vi "Measurement UI.vi"() -> ()   [LabVIEW 2021, in "Efficiency_Channel Ganging_UI.lvlib"]
uses:
  Efficiency_Channel Ganging_UI.lvlib
panel:
  in  "MeasGraphs":enum32{"Efficiency", "Hidden Controls"}(tab)
  out "EfficiencyGraph":T1(graph)
  in  "Load current pole-zero ratios":dbl[](array[numeric])
  in  "Load current compensation frequencies":dbl[](array[numeric])
  in  "Load current gain bandwidths":dbl[](array[numeric])
  in  "Source voltage pole-zero ratios":dbl[](array[numeric])
  in  "Source voltage compensation frequencies":dbl[](array[numeric])
  in  "Source voltage gain bandwidths":dbl[](array[numeric])
  in  "Load slave resource names":string[](array[string])
  in  "Load master resource name":string
  in  "Source slave resource names":string[](array[string])
  in  "Source master resource name":string
  out "Load sweep points":i32
  out "Source sweep points":i32
  out "Voltage values":dbl[](array[numeric])
  out "Efficiency":dbl[](array[numeric])
  out "Ganged load currents":dbl[](array[numeric])
  in  "MeasConfigurations":T2(tab)=enum."Source Config"
  in  "Source delay":dbl=0.005 caption="SOURCE DELAY" format="%.3ps"
  in  "DUT setup time":dbl=1.0 caption="DUT SETUP TIME" format="%.3ps"
  in  "Aperture time":dbl=0.005 caption="APERTURE TIME" format="%.3ps"
  in  "PPSSlaveResourceNames":refnum<k15>[](array[refnum]) caption="SLAVE RESOURCE NAMES"
  in  "PPSMasterResourceName":refnum<k15> caption="MASTER RESOURCE NAME"
  in  "Source stop voltage":dbl=14.0 caption="VOLTAGE STOP LEVEL" format="%#_6pV"
  in  "Source transient response":i32(ring)=1038 caption="TRANSIENT RESPONSE" items=["Slow"=1041, "Normal"=1038, "Fast"=1039, "Custom"=1042]
  in  "Source sense":i32(ring)=1009 caption="SENSE" items=["Local"=1008, "Remote"=1009]
  in  "Source voltage level range":dbl=20.0 caption="VOLTAGE LEVEL RANGE" format="%#_6pV"
  in  "Source start voltage":dbl=6.0 caption="VOLTAGE START LEVEL" format="%#_6pV"
  in  "Source current limit high":dbl=25.0 caption="CURRENT LIMIT/LIMIT HIGH" format="%#_6pA"
  in  "Source current limit range":dbl=25.0 caption="CURRENT LIMIT RANGE" format="%#_6pA"
  in  "Source limit symmetry":enum32{"Symmetric", "Asymmetric"}(ring)=enum."Asymmetric" caption="LIMIT SYMMETRY"
  in  "Source current limit low":dbl=-0.6 caption="CURRENT LIMIT LOW" format="%#_6pA"
  in  "Source system configuration":enum32{"Series", "Parallel"}(ring)=enum."Parallel" caption="SYSTEM CONFIG"
  in  "Source compliance":string="Compliance"
  in  "Source sourceadapt":string="SourceAdapt"
  in  "Source voltage sweep points":i32=4 caption="NO. OF POINTS"
  in  "Source Custom Transient Response":bool
  in  "Load current sweep points/points per decade":i32=10 caption="PTS/PTS PER DECADE"
  in  "Load sweep type":string(combo)="Logarithmic" caption="SWEEP TYPE"
  in  "Load stop current":dbl=50.0 caption="CURRENT STOP LEVEL" format="%#_6pA"
  in  "Load sourceadapt":string="SourceAdapt"
  in  "Load compliance":string="Compliance"
  in  "Load system configuration":enum32{"Series", "Parallel"}(ring)=enum."Parallel" caption="SYSTEM CONFIG"
  in  "Load voltage limit low":dbl caption="VOLTAGE  LIMIT LOW" format="%#_6pV"
  in  "Load limit symmetry":enum32{"Symmetric", "Asymmetric"}(ring) caption="LIMIT SYMMETRY"
  in  "Load voltage limit range":dbl=6.0 caption="VOLTAGE LIMIT RANGE" format="%#_6pV"
  in  "Load voltage limit high":dbl=inf caption="VOLTAGE LIMIT/LIMIT HIGH" format="%#_6p"
  in  "Load start current":dbl=2.0 caption="CURRENT START LEVEL" format="%#_6pA"
  in  "Load current level range":dbl=80.0 caption="CURRENT LEVEL RANGE" format="%#_6pA"
  in  "Load sense":i32(ring)=1009 caption="SENSE" items=["Local"=1008, "Remote"=1009]
  in  "Load transient response":i32(ring)=1038 caption="TRANSIENT RESPONSE" items=["Slow"=1041, "Normal"=1038, "Fast"=1039, "Custom"=1042]
  in  "LoadSlaveResourceNames":refnum<k15>[](array[refnum]) caption="SLAVE RESOURCE NAMES"
  in  "LoadMasterResourceName":refnum<k15> caption="MASTER RESOURCE NAME"
  in  "Load Custom Transient Response":bool
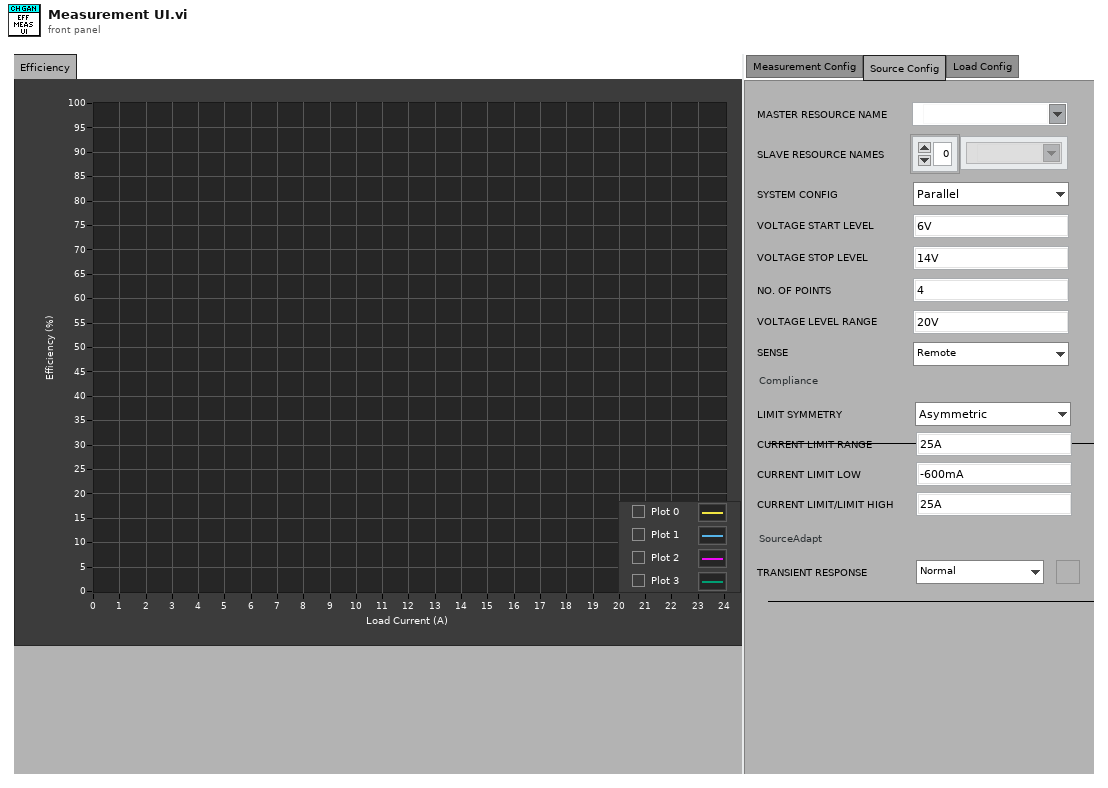
[diagram p1: front panel]
types:
  T1 = cluster{"Ganged load currents":dbl[], "Efficiency":dbl[]}[]
  T2 = enum32{"Measurement Config", "Source Config", "Load Config"}
  T3 = typedef "SourceAdapt Parameters.ctl" = cluster{"Voltage gain bandwidth":dbl, "Voltage compensation frequency":dbl, "Voltage pole-zero ratio":dbl, "Current gain bandwidth":dbl, "Current compensation frequency":dbl, "Current pole-zero ratio":dbl}[]
  T4 = cluster{"Ganged load currents":dbl[], "Efficiency":dbl[]}
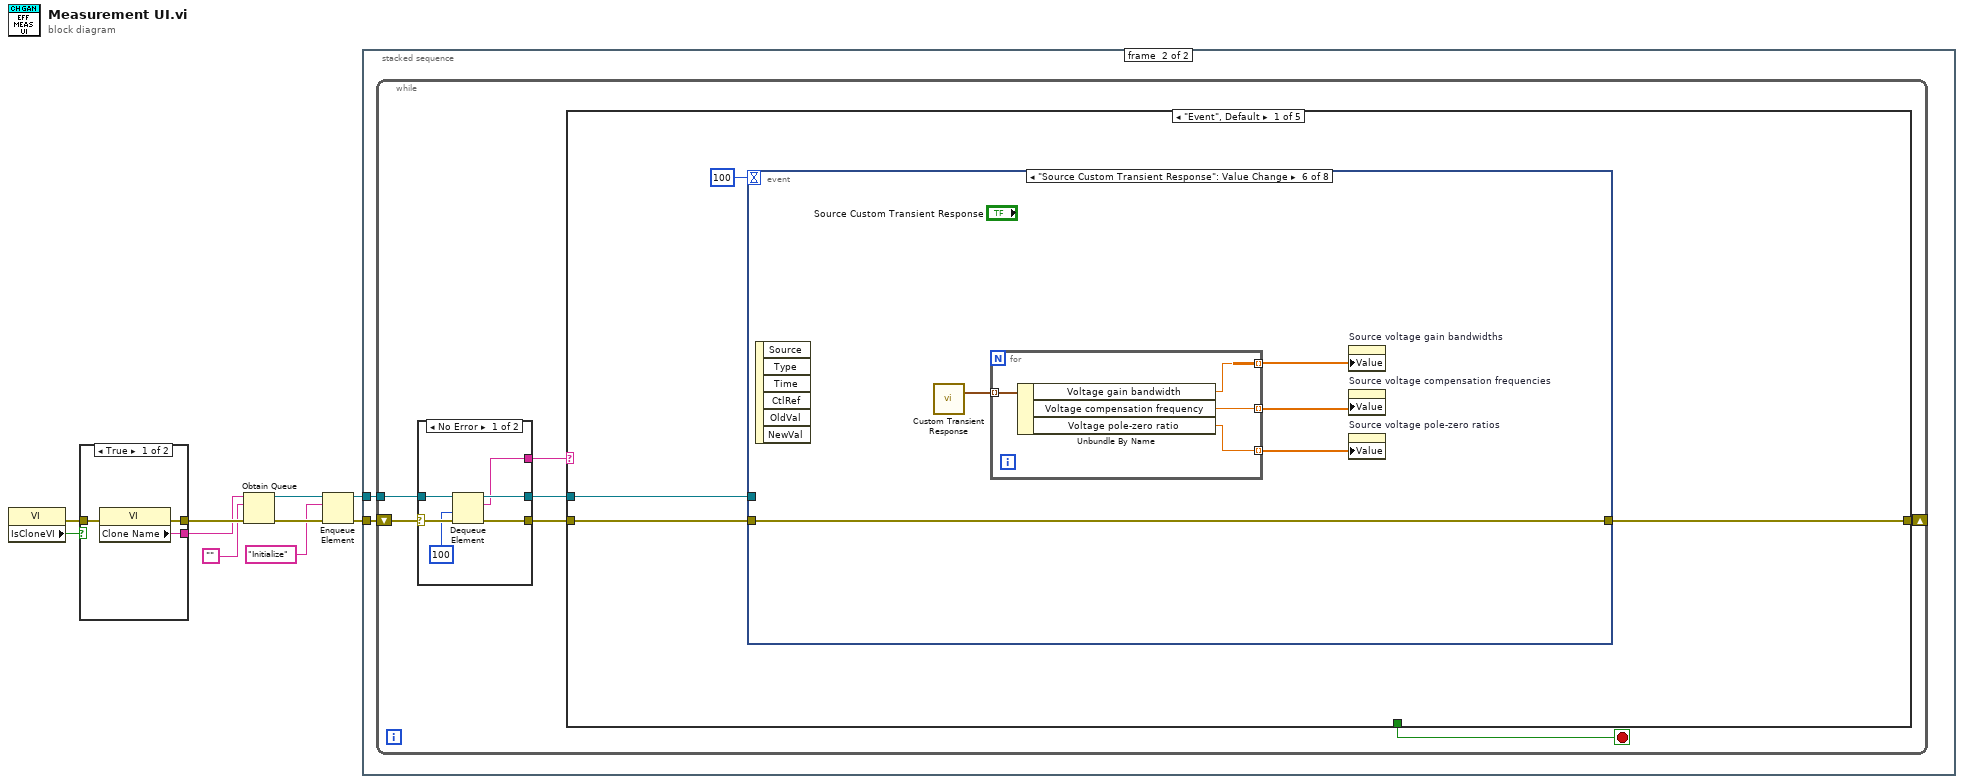
[diagram p0: block diagram]
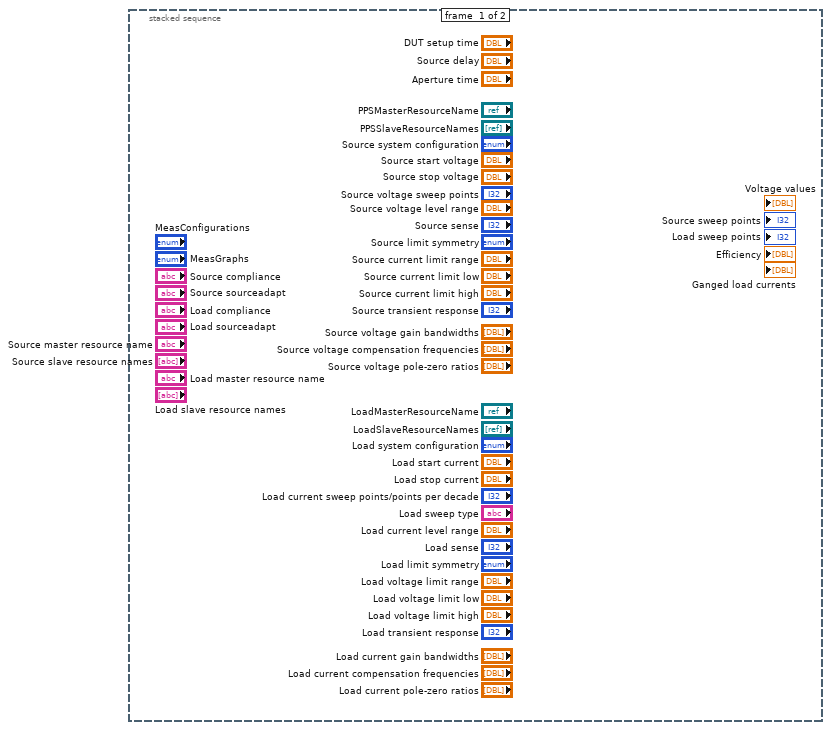
[diagram p2: hidden frame]
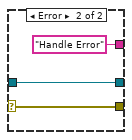
[diagram p3: hidden frame]
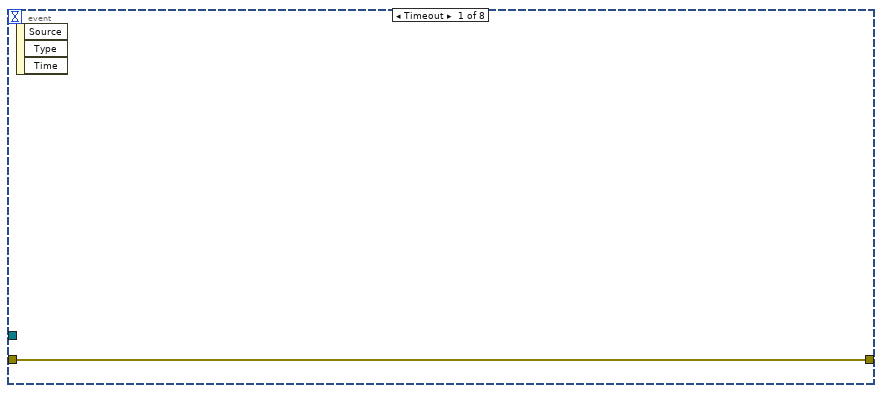
[diagram p4: hidden frame]
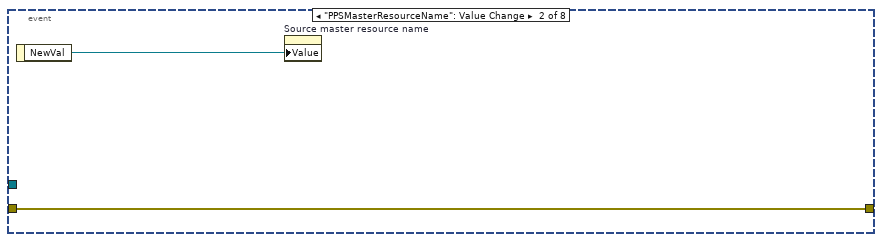
[diagram p5: hidden frame]
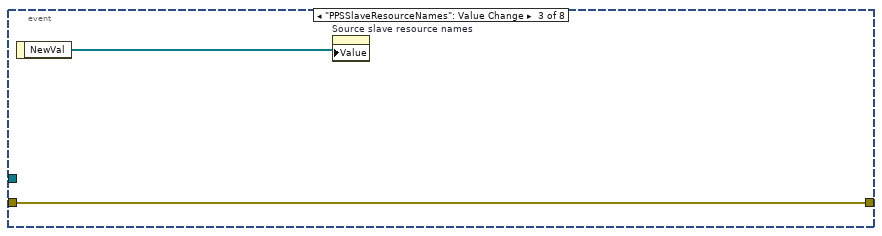
[diagram p6: hidden frame]
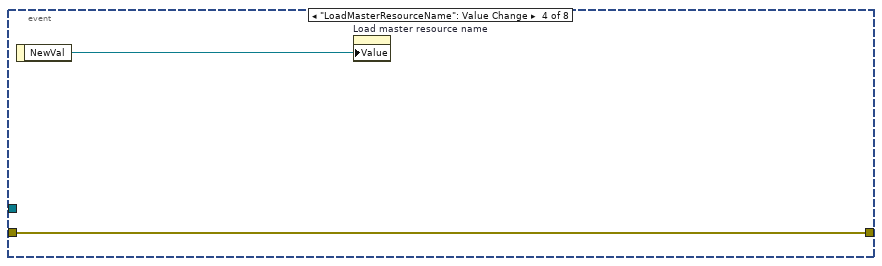
[diagram p7: hidden frame]
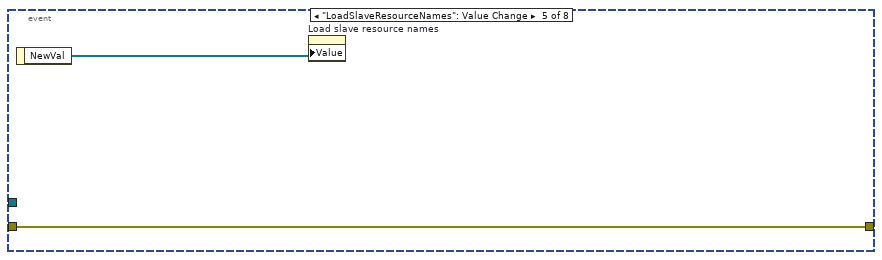
[diagram p8: hidden frame]
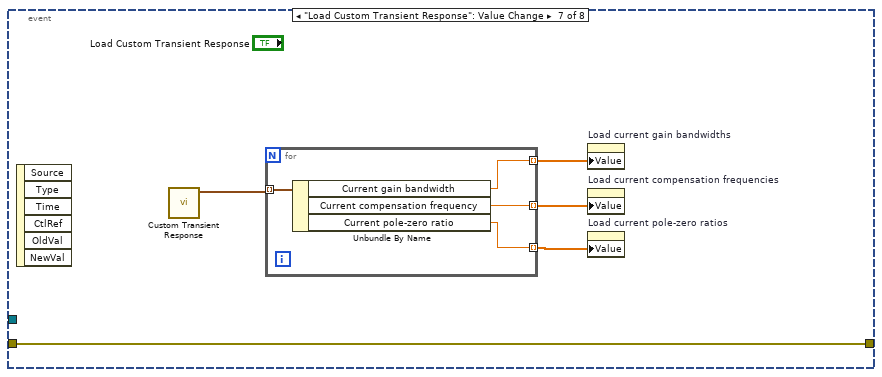
[diagram p9: hidden frame]
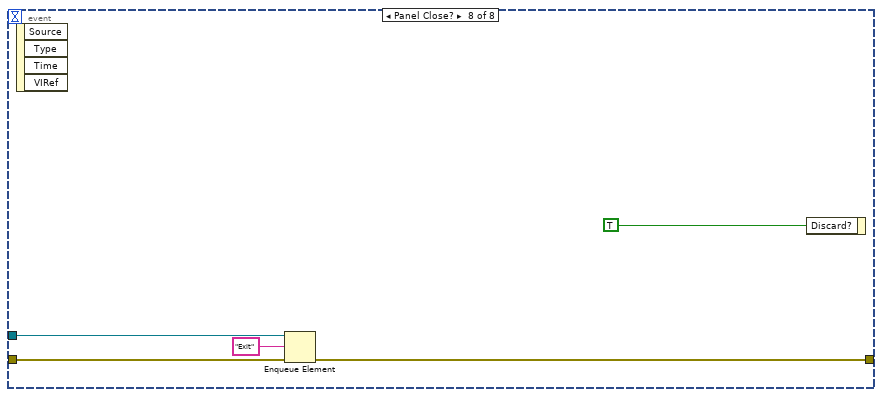
[diagram p10: hidden frame]
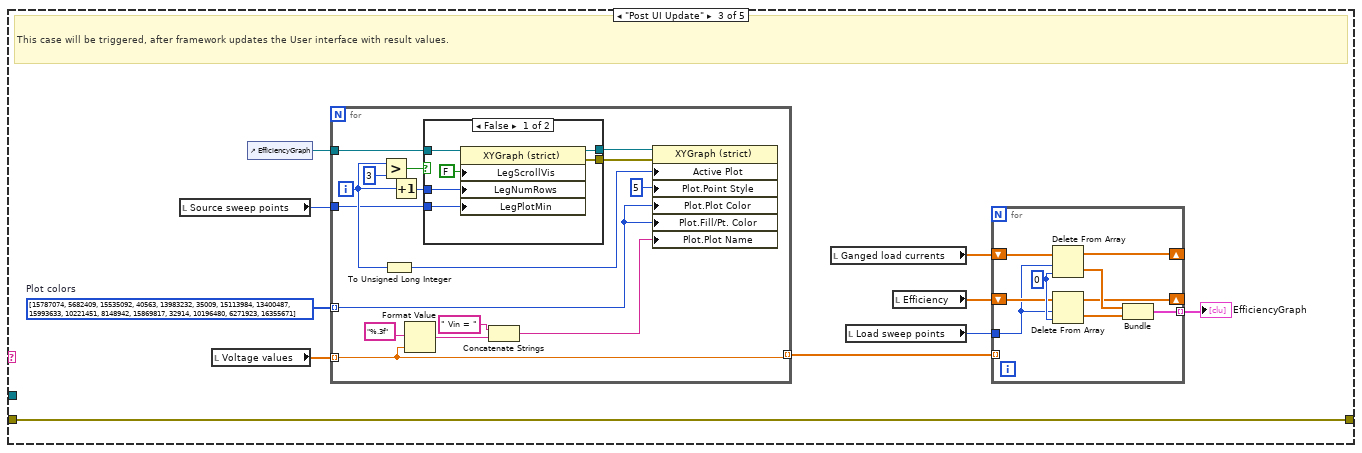
[diagram p12: hidden frame]
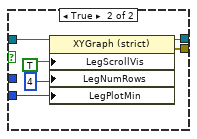
[diagram p13: hidden frame]
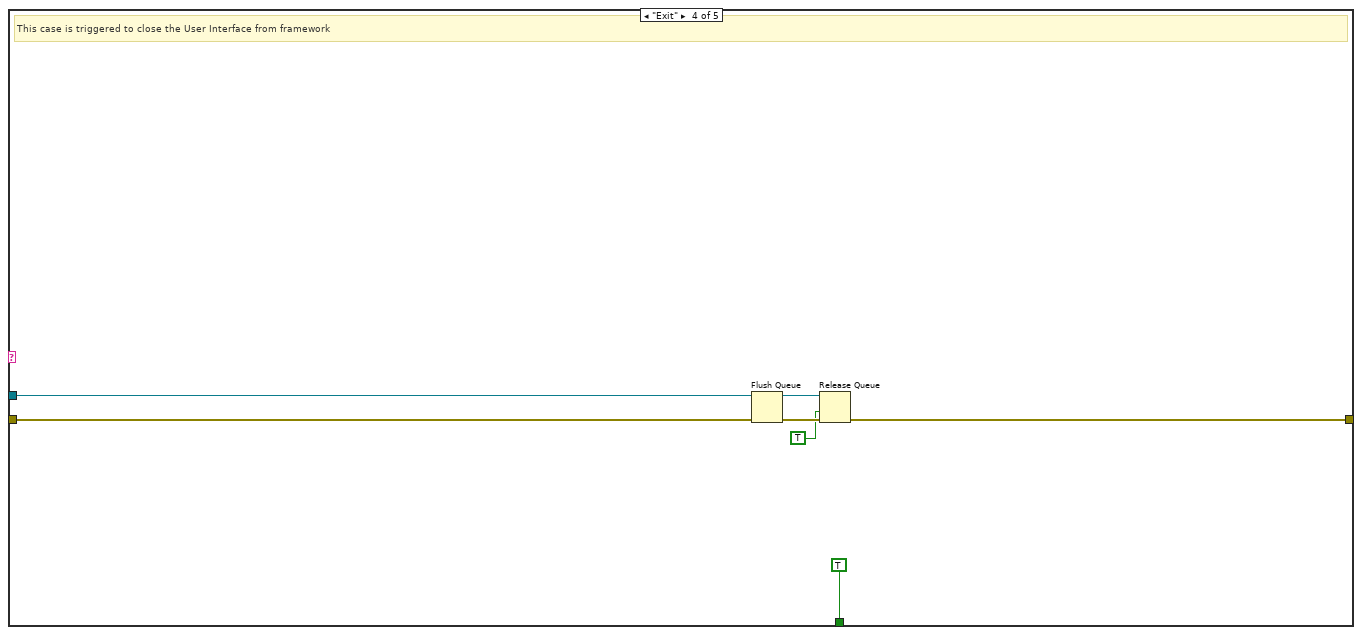
[diagram p14: hidden frame]
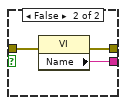
[diagram p16: hidden frame]
diagram:
  n1 = property class="VI"() -> (error out=w1:errorcluster, "IsCloneVI"=w2:bool)  [unwired: 2 in, 1 out]
  n2 = case shown="True" w2 {
    tunnel: [w13 w16] -> w10
    tunnel: [w12 w15] -> w9
    tunnel: w1 -> [w11 w14]
    frame True {
      n3 = property class="VI"(error in=w11) -> (error out=w13:errorcluster, "Clone Name"=w12:string)  [unwired: 1 in, 1 out]
    }
    frame False {
      n4 = property class="VI"(error in=w14) -> (error out=w16:errorcluster, "Name"=w15:string)  [unwired: 1 in, 1 out]
    }
  }
  n5 = Obtain Queue(name (unnamed)=w9, element data type="", error in (no error)=w10) -> (queue out=w6:refnum<queue>, error out=w8:errorcluster)  [unwired: 2 in, 1 out]
  n6 = Enqueue Element(queue=w6, element="Initialize", error in (no error)=w8) -> (queue out=w5:refnum<queue>, error out=w7:errorcluster)  [unwired: 1 in, 1 out]
  n7 = stacked-sequence {
    tunnel: w7 -> [_ w18]
    tunnel: w5 -> [_ w17]
    frame #0 {
    }
    frame #1 {
      n8 = while {
        shift-right: [w20] -> _
        shift-left: w18 -> [w25]
        tunnel: w17 -> [w23]
        stop <- w19 stop-if-true
        n9 = case shown="No Error" w25 {
          selector: w25 -> [w31 w34]
          tunnel: [w30 w34] -> w24
          tunnel: w23 -> [w29 w33]
          tunnel: [w28 w33] -> w22
          tunnel: [w27 "Handle Error"] -> w21
          frame No Error {
            n10 = Dequeue Element(queue=w29, timeout in ms (-1)=100, error in (no error)=w31) -> (queue out=w28:refnum<queue>, element=w27:string, error out=w30:errorcluster)  [unwired: 1 out]
          }
          frame Error {
          }
        }
        n11 = case shown="\"Event\", Default" w21 {
          tunnel: w24 -> [w37 w71 w81 w125 w126]
          tunnel: w22 -> [w35 _ _ w123 _]
          tunnel: [w38 w71 w81 w120 w126] -> w20
          tunnel: [_ _ _ TRUE _] -> w19
          frame "Event", Default {
            n12 = event shown="[5] \"Source Custom Transient Response\": Value Change" {
              selector: _ -> [_ _ _ _ _ _ _ _]
              dyn-events: _ -> [_ _ _ _ _ _ _ _]
              timeout: 100 -> [_ _ _ _ _ _ _ _]
              tunnel: [w39 w41 w43 w44 w46 w48 w57 w68] -> w38
              tunnel: w37 -> [w39 w41 w43 w44 w46 w48 w57 w69]
              tunnel: w35 -> [_ _ _ _ _ _ _ w67]
              event Timeout {
                n13 = event-data() -> ()  [unwired: 1 in, 3 out]
              }
              event "PPSMasterResourceName": Value Change {
                n14 = event-data() -> ("NewVal"=w40:refnum<k15>)  [unwired: 1 in]
                n15 = property on="Source master resource name" class="Str"("Value"=w40) -> ()  [unwired: 2 in, 2 out]
              }
              event "PPSSlaveResourceNames": Value Change {
                n16 = event-data() -> ("NewVal"=w42:refnum<k15>[])  [unwired: 1 in]
                n17 = property on="Source slave resource names" class="Arr (strict)"("Value"=w42) -> ()  [unwired: 2 in, 2 out]
              }
              event "LoadMasterResourceName": Value Change {
                n18 = event-data() -> ("NewVal"=w45:refnum<k15>)  [unwired: 1 in]
                n19 = property on="Load master resource name" class="Str"("Value"=w45) -> ()  [unwired: 2 in, 2 out]
              }
              event "LoadSlaveResourceNames": Value Change {
                n20 = event-data() -> ("NewVal"=w47:refnum<k15>[])  [unwired: 1 in]
                n21 = property on="Load slave resource names" class="Arr (strict)"("Value"=w47) -> ()  [unwired: 2 in, 2 out]
              }
              event "Source Custom Transient Response": Value Change {
                n22 = event-data() -> ()  [unwired: 1 in, 6 out]
                n23 = call "Custom Transient Response.vi"() -> ("SourceAdapt Parameters"=w52:T3)  [unwired: 11 in]
                n24 = for {
                  tunnel: w52 -> [w56] mode=indexing
                  tunnel: [w55] -> w51 mode=indexing
                  tunnel: [w54] -> w50 mode=indexing
                  tunnel: [w53] -> w49 mode=indexing
                  n25 = Unbundle By Name(w56) -> ("Voltage gain bandwidth"=w55:dbl, "Voltage compensation frequency"=w54:dbl, "Voltage pole-zero ratio"=w53:dbl)
                }
                n26 = property on="Source voltage gain bandwidths" class="Arr (strict)"("Value"=w51) -> ()  [unwired: 2 in, 2 out]
                n27 = property on="Source voltage compensation frequencies" class="Arr (strict)"("Value"=w50) -> ()  [unwired: 2 in, 2 out]
                n28 = property on="Source voltage pole-zero ratios" class="Arr (strict)"("Value"=w49) -> ()  [unwired: 2 in, 2 out]
              }
              event "Load Custom Transient Response": Value Change {
                n29 = event-data() -> ()  [unwired: 1 in, 6 out]
                n30 = call "Custom Transient Response.vi"() -> ("SourceAdapt Parameters"=w61:T3)  [unwired: 11 in]
                n31 = for {
                  tunnel: w61 -> [w65] mode=indexing
                  tunnel: [w64] -> w60 mode=indexing
                  tunnel: [w63] -> w59 mode=indexing
                  tunnel: [w62] -> w58 mode=indexing
                  n32 = Unbundle By Name(w65) -> ("Current gain bandwidth"=w64:dbl, "Current compensation frequency"=w63:dbl, "Current pole-zero ratio"=w62:dbl)
                }
                n33 = property on="Load current gain bandwidths" class="Arr (strict)"("Value"=w60) -> ()  [unwired: 2 in, 2 out]
                n34 = property on="Load current compensation frequencies" class="Arr (strict)"("Value"=w59) -> ()  [unwired: 2 in, 2 out]
                n35 = property on="Load current pole-zero ratios" class="Arr (strict)"("Value"=w58) -> ()  [unwired: 2 in, 2 out]
              }
              event Panel Close? {
                n36 = event-data() -> ()  [unwired: 1 in, 4 out]
                n37 = Enqueue Element(queue=w67, element="Exit", error in (no error)=w69) -> (error out=w68:errorcluster)  [unwired: 1 in, 2 out]
                n38 = event-data("Discard?"=TRUE) -> ()  [unwired: 1 in, 1 out]
              }
            }
          }
          frame "Initialize" {
          }
          frame "Post UI Update" {
            w76 = u32[] [15787074, 5682409, 15535092, 40563, 13983232, 35009, 15113984, 13400487, 15993633, 10221451, 8148942, 15869817, 32914, 10196480, 6271923, 16355671]  # Plot colors
            # "This case will be triggered, after framework updates the User interface with result values."
            n39 = local read "Source sweep points"() -> (w73:i32)
            n40 = local read "Voltage values"() -> (w74:dbl[])
            n41 = control-ref of="EfficiencyGraph"() -> (w75:refnum<vi>)
            n42 = for {
              tunnel: w74 -> [w94] mode=indexing
              tunnel: [w94] -> w72 mode=indexing
              tunnel: w75 -> [w87]
              tunnel: w73 -> [w84]
              tunnel: w76 -> [w90] mode=indexing
              i -> [w88]
              n43 = Greater?(x=w88, y=3) -> (0:w92:bool)
              n44 = To Unsigned Long Integer(number=w88) -> (unsigned 32bit integer=w91:u32)
              n45 = Increment(x=w88) -> (x+1=w86:i32)
              n46 = Format Value(format string="%.3f", value (0)=w94) -> (output string=w97:string)  [unwired: 1 out]
              n47 = case shown="False" w92 {
                tunnel: w87 -> [w103 w109]
                tunnel: w86 -> [w102 _]
                tunnel: [w101 w108] -> w85
                tunnel: w84 -> [w99 w104]
                tunnel: [w100 w107] -> w83
                frame False {
                  n48 = property on="Property Node" class="XYGraph (strict)"(reference=w103, "LegScrollVis"=FALSE ("Legend:Scrollbar Visible"), "LegNumRows"=w102, "LegPlotMin"=w99) -> (reference out=w101:refnum<vi>, error out=w100:errorcluster)  [unwired: 1 in]
                }
                frame True {
                  n49 = property on="Property Node" class="XYGraph (strict)"(reference=w109, "LegScrollVis"=TRUE ("Legend:Scrollbar Visible"), "LegNumRows"=u32 4 ("Legend:Number of Rows"), "LegPlotMin"=w104) -> (reference out=w108:refnum<vi>, error out=w107:errorcluster)  [unwired: 1 in]
                }
              }
              n50 = Concatenate Strings(" Vin = " ("string"), w97) -> (w82:string)
              n51 = property on="Property Node" class="XYGraph (strict)"(reference=w85, error in=w83, "Active Plot"=w91, "Plot.Point Style"=u8 5, "Plot.Plot Color"=w90, "Plot.Fill/Pt. Color"=w90, "Plot.Plot Name"=w82) -> ()  [unwired: 2 out]
            }
            n52 = local read "Ganged load currents"() -> (w80:dbl[])
            n53 = local read "Load sweep points"() -> (w77:i32)
            n54 = local read "Efficiency"() -> (w79:dbl[])
            n55 = for {
              tunnel: [w118] -> w78 mode=indexing
              shift-right: [w117] -> _
              shift-left: w80 -> [w113]
              shift-right: [w111] -> _
              shift-left: w79 -> [w112]
              tunnel: w77 -> [w110]
              tunnel: w72 -> [_] mode=indexing
              w114 = 0 ("index")
              n56 = Delete From Array(array=w113, length=w110, index=w114) -> (deleted portion=w116:dbl[], array with subset deleted=w117:dbl[])
              n57 = Delete From Array(array=w112, length=w110, index=w114) -> (deleted portion=w115:dbl[], array with subset deleted=w111:dbl[])
              n58 = Bundle("Ganged load currents"=w116, "Efficiency"=w115) -> (w118:T4)  [unwired: 1 in]
            }
            "EfficiencyGraph" <- w78
          }
          frame "Exit" {
            # "This case is triggered to close the User Interface from framework"
            n59 = Flush Queue(queue=w123, error in (no error)=w125) -> (queue out=w122:refnum<queue>, error out=w121:errorcluster)  [unwired: 1 out]
            n60 = Release Queue(queue=w122, force destroy? (F)=TRUE, error in (no error)=w121) -> (error out=w120:errorcluster)  [unwired: 2 out]
          }
          frame "Handle Error" {
          }
        }
      }
    }
  }
